vi "ODH_LEGO_Consumer.vi"() -> ()   [LabVIEW 2016]
uses:
  Controls/Lego_State_Control.ctl
  Controls/Lego_ComboBox_Parameters.ctl
  <vilib>/NXT/Block Support/NXT_OutputPort.ctl
  <vilib>/NXT/NXTIO Xnodes/NXTIONodeSubVIs/NXTMotorRunDistance.vi
  <vilib>/NXT/NXTIO Xnodes/AddressXNode/NXTIOAddress.xnode
  <vilib>/NXT/Subs/LVHSConnector.ctl
  <vilib>/NXT/NXTIO Xnodes/NXTIOXNode/NXTIO.xnode
  <vilib>/NXT/LegoClasses/BrickReference/BrickReference.lvclass
panel:
  out "Current State":T1
  out "Error Out":errorcluster
  in  "Error In":errorcluster
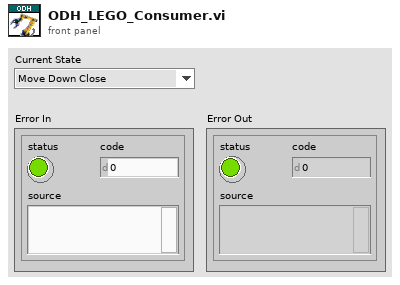
[diagram p1: front panel]
types:
  T1 = typedef "Lego_State_Control.ctl" = enum16{"Move Down Close", "Move Down Open", "Move Down Comfort Close", "Move Up Open", "Move Up Close", "Move Up Comfort Close", "Wait"}
  T2 = typedef "Lego_ComboBox_Parameters.ctl" = string
  T3 = typedef "NXT_OutputPort.ctl" = u8
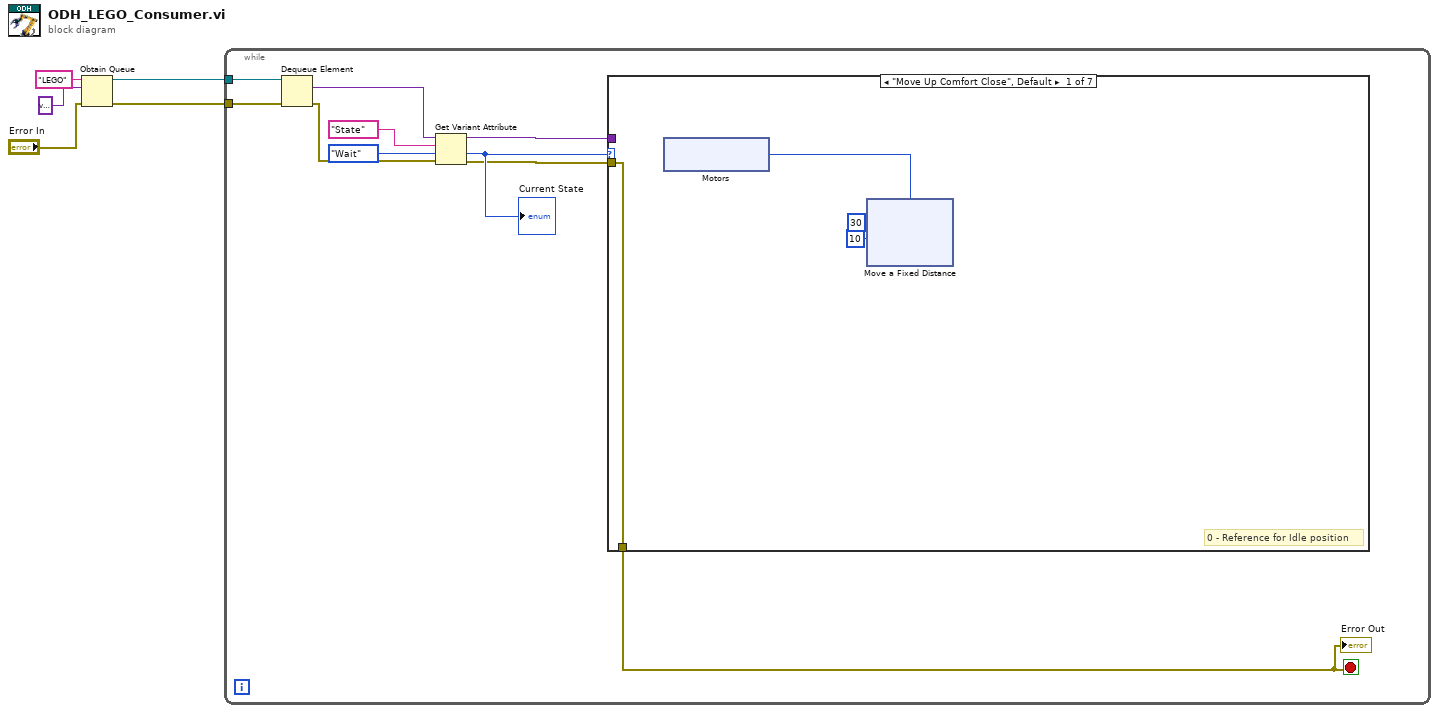
[diagram p0: block diagram]
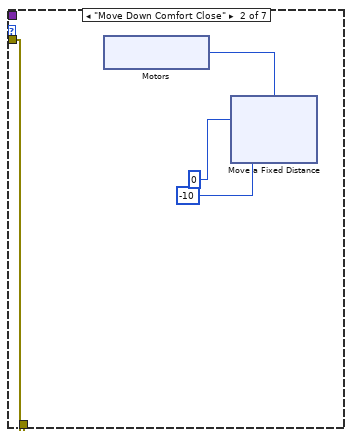
[diagram p2: hidden frame]
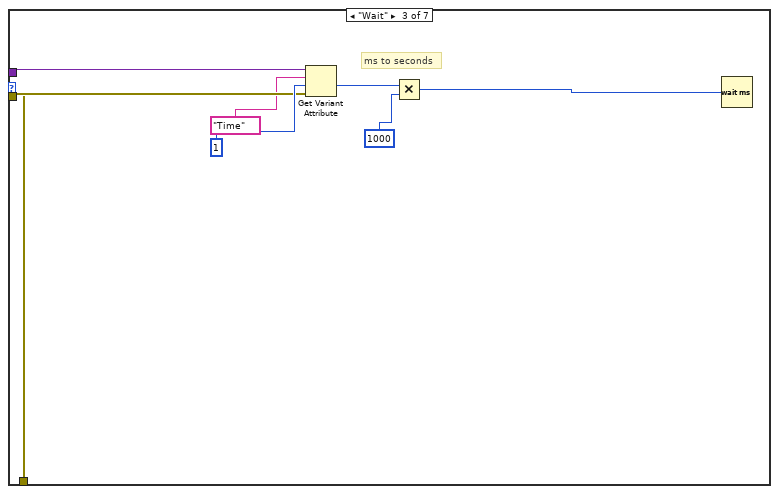
[diagram p3: hidden frame]
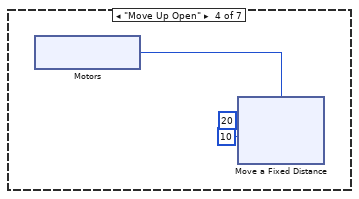
[diagram p4: hidden frame]
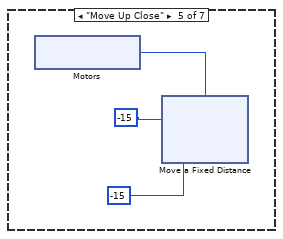
[diagram p5: hidden frame]
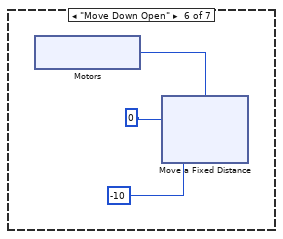
[diagram p6: hidden frame]
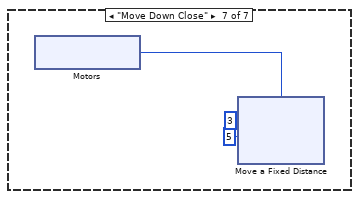
[diagram p7: hidden frame]
diagram:
  n1 = Obtain Queue(name (unnamed)="LEGO", element data type=variant, error in (no error)="Error In") -> (queue out=w4:refnum<queue>, error out=w5:errorcluster)  [unwired: 2 in, 1 out]
  n2 = while {
    tunnel: w5 -> [w15]
    tunnel: w4 -> [w14]
    stop <- w6 stop-if-true
    n3 = Dequeue Element(queue=w14, error in (no error)=w15) -> (element=w13:variant, error out=w9:errorcluster)  [unwired: 1 in, 2 out]
    n4 = Get Variant Attribute(Variant=w13, name=T2 "State" ("Combo Box"), default value (empty Variant)=Lego_State_Control."Wait" ("Enum"), error in=w9) -> (duplicate Variant=w10:variant, value=w12:T1, error out=w8:errorcluster)  [unwired: 1 out]
    "Current State" <- w12
    n5 = case shown="\"Move Up Comfort Close\", Default" w12 {
      tunnel: w10 -> [_ _ w53 _ _ _ _]
      tunnel: w8 -> [w19 w34 w51 _ _ _ _]
      tunnel: [w19 w34 w50 _ _ _ _] -> w6
      frame "Move Up Comfort Close", Default {
        # "0 - Reference for Idle position"
        n6 = xnode "Motors"() -> ("Motor"=w16:T3)
        n7 = xnode "Move a Fixed Distance"("Speed 1"=i8 10, "Distance 1"=30, "Motors"=w16) -> ()  [unwired: 1 in, 1 out]
      }
      frame "Move Down Comfort Close" {
        n8 = xnode "Motors"() -> ("Motor"=w31:T3)
        n9 = xnode "Move a Fixed Distance"("Speed 1"=i8 -10, "Distance 1"=0, "Motors"=w31) -> ()  [unwired: 1 in, 1 out]
      }
      frame "Wait" {
        # "ms to seconds"
        n10 = Get Variant Attribute(Variant=w53, name=T2 "Time" ("Combo Box"), default value (empty Variant)=1, error in=w51) -> (value=w48:i32, error out=w50:errorcluster)  [unwired: 2 out]
        n11 = Multiply(x=w48, y=1000) -> (x*y=w46:i32)
        n12 = Wait (ms)(milliseconds to wait=w46) -> ()  [unwired: 1 out]
      }
      frame "Move Up Open" {
        n13 = xnode "Motors"() -> ("Motor"=w54:T3)
        n14 = xnode "Move a Fixed Distance"("Speed 1"=i8 10, "Distance 1"=20, "Motors"=w54) -> ()  [unwired: 1 in, 1 out]
      }
      frame "Move Up Close" {
        n15 = xnode "Motors"() -> ("Motor"=w68:T3)
        n16 = xnode "Move a Fixed Distance"("Speed 1"=i8 -15, "Distance 1"=-15, "Motors"=w68) -> ()  [unwired: 1 in, 1 out]
      }
      frame "Move Down Open" {
        n17 = xnode "Motors"() -> ("Motor"=w82:T3)
        n18 = xnode "Move a Fixed Distance"("Speed 1"=i8 -10, "Distance 1"=0, "Motors"=w82) -> ()  [unwired: 1 in, 1 out]
      }
      frame "Move Down Close" {
        n19 = xnode "Motors"() -> ("Motor"=w96:T3)
        n20 = xnode "Move a Fixed Distance"("Speed 1"=i8 5, "Distance 1"=3, "Motors"=w96) -> ()  [unwired: 1 in, 1 out]
      }
    }
    "Error Out" <- w6
  }
